vi "AddDateToFile.vi"(8 "error in (no error)":errorcluster, 11 "file name":string) -> (0 "error out":errorcluster, 3 "new file path (Not A Path if cancelled)":path)   [LabVIEW 2019]
uses:
  <vilib>/Utility/file.llb/Write Delimited Spreadsheet (string).vi
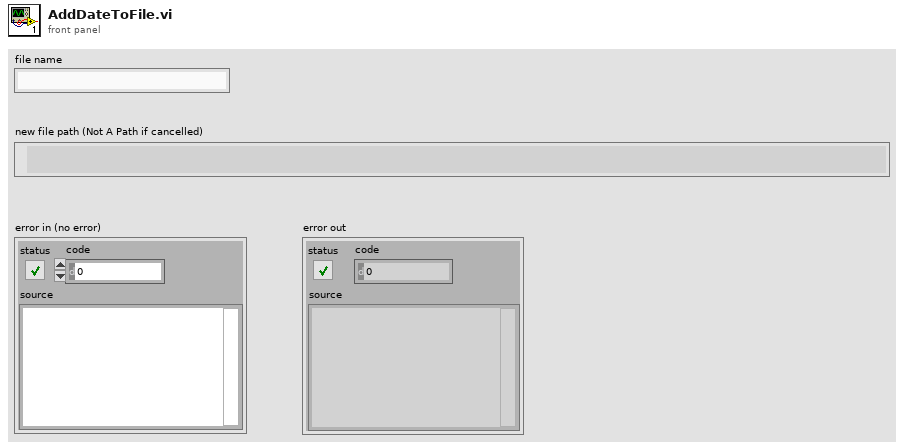
[diagram p1: front panel]
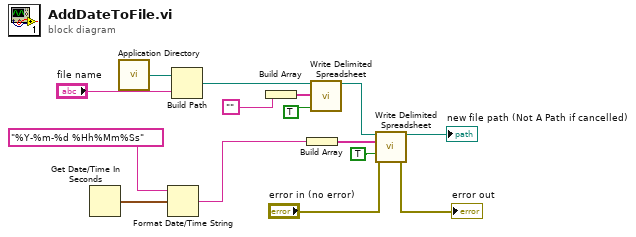
[diagram p0: block diagram]
diagram:
  n1 = Get Date/Time In Seconds() -> (seconds since 1Jan1904=w15:timestamp)
  n2 = call <vilib>:"Application Directory.vi"() -> ("Application Directory"=w4:path)
  n3 = Format Date/Time String(time format string (%c)="%Y-%m-%d %Hh%Mm%Ss" ("date/time string"), seconds (now)=w15) -> (date/time string=w2:string)  [unwired: 1 in]
  n4 = Build Path(base path=w4, name or relative path="file name") -> (appended path=w5:path)
  n5 = Build Array("") -> (w10:string[])
  n6 = Build Array(w2) -> (w13:string[])
  n7 = call-poly <vilib>:"Write Delimited Spreadsheet.vi"("file path (dialog if empty)"=w5, "1D data"=w10, "append to file? (new file:F)"=TRUE) -> ("new file path (Not A Path if cancelled)"=w9:path)  [unwired: 11 in, 1 out]
  n8 = call-poly <vilib>:"Write Delimited Spreadsheet.vi"("file path (dialog if empty)"=w9, "1D data"=w13, "append to file? (new file:F)"=TRUE, "error in (no error)"="error in (no error)") -> ("new file path (Not A Path if cancelled)"=→"new file path (Not A Path if cancelled)":path, "error out"=→"error out":errorcluster)  [unwired: 10 in]
